vi "Setup DCPower Current for ELOAD.vi"(7 "Channel Groups?":bool, 8 "error in":errorcluster, 9 "Parameters":T1={"Supply"=0.0, "Limit"=0.0, "Aperture Time"=0.0, "Settling Time"=0.0, "Sense"=1008, "Transient Response"=1041} {"Transient Response" items=["Slow"=1041, "Normal"=1038, "Fast"=1039, "Custom"=1042]; "Sense" items=["Local"=1008, "Remote"=1009]}, 10 "Channel List":string, 11 "DCPower Handle In":refnum<k15>) -> (0 "error out":errorcluster, 3 "DCPower Handle Out":refnum<k15>)   [LabVIEW 2021, in "PMIC Common.lvlib"]
uses:
  PMIC Common.lvlib
  DCPower Parameters.ctl
  <instrlib>/niDCPower/nidcpower.llb/niDCPower Output Function.ctl
  <instrlib>/niDCPower/nidcpower.llb/niDCPower Source Mode.ctl
  <instrlib>/niDCPower/nidcpower.llb/niDCPower Wait For Event - Event.ctl
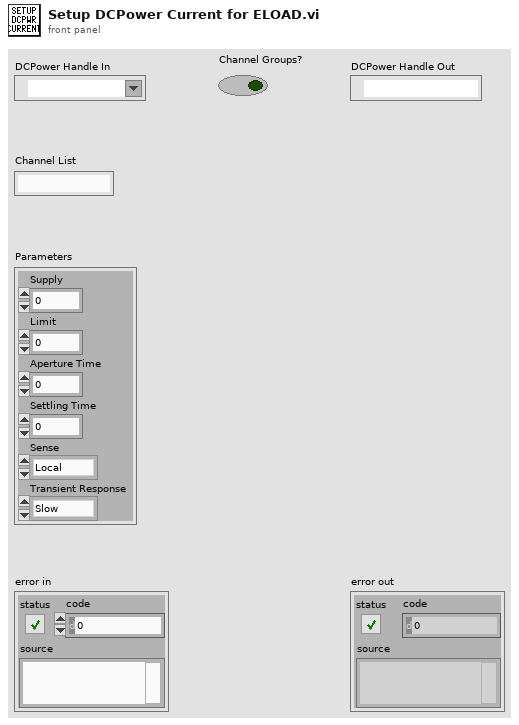
[diagram p1: front panel]
types:
  T1 = typedef "PMIC Common.lvlib/DCPower Parameters.ctl" = cluster{"Supply":dbl, "Limit":dbl, "Aperture Time":dbl, "Settling Time":dbl, "Sense":i32, "Transient Response":i32}
  T2 = typedef "niDCPower Source Mode.ctl" = i32
  T3 = typedef "niDCPower Output Function.ctl" = i32
  T4 = typedef "niDCPower Wait For Event - Event.ctl" = i32
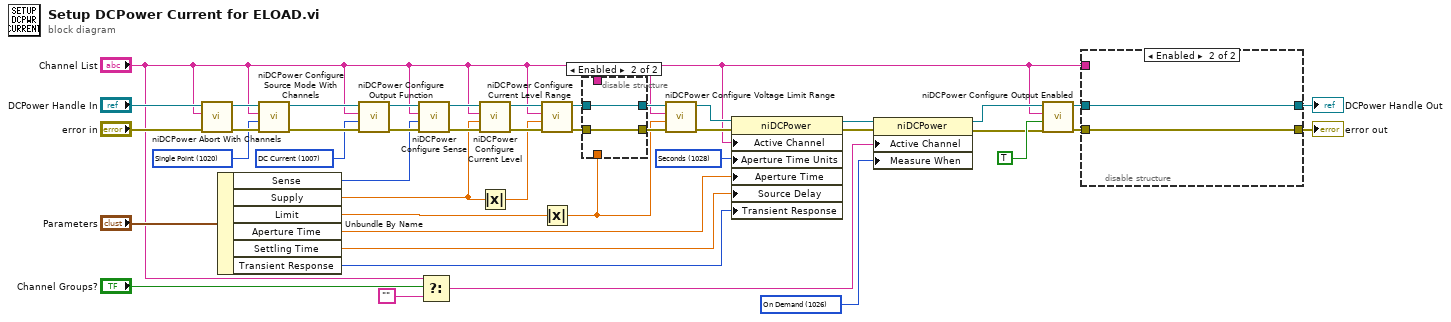
[diagram p0: block diagram]
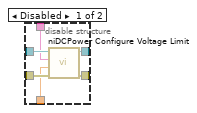
[diagram p2: hidden frame]
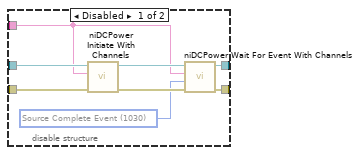
[diagram p3: hidden frame]
diagram:
  w15 = 1026 items=["Automatically after Source Complete"=1025, "On Demand"=1026, "On Measure Trigger"=1027] ("Measurement:Advanced:Measure When")
  w31 = T2 1020 items=["Single Point"=1020, "Sequence"=1021] ("source mode")
  w35 = 1028 items=["Seconds"=1028, "Power Line Cycles"=1029] ("Measurement:Aperture Time Units")
  w1 = T3 1007 items=["DC Voltage"=1006, "DC Current"=1007, "Pulse Voltage"=1049, "Pulse Current"=1050] ("output function")
  n1 = call <instrlib>:"niDCPower Abort With Channels.vi"("error in (no error)"="error in", "channel name"="Channel List", "instrument handle"="DCPower Handle In") -> ("error out"=w33:errorcluster, "instrument handle out"=w44:refnum<k15>)  [unwired: 7 in]
  n2 = Unbundle By Name("Parameters") -> ("Sense"=w8:i32, "Supply"=w7:dbl, "Limit"=w6:dbl, "Aperture Time"=w5:dbl, "Settling Time"=w4:dbl, "Transient Response"=w3:i32)
  n3 = call <instrlib>:"niDCPower Configure Source Mode With Channels.vi"("error in (no error)"=w33, "source mode"=w31, "channel name"="Channel List", "instrument handle"=w44) -> ("error out"=w32:errorcluster, "instrument handle out"=w34:refnum<k15>)  [unwired: 6 in]
  n4 = call <instrlib>:"niDCPower Configure Output Function.vi"("error in (no error)"=w32, "output function"=w1, "channel name"="Channel List", "instrument handle"=w34) -> ("error out"=w26:errorcluster, "instrument handle out"=w25:refnum<k15>)  [unwired: 6 in]
  n5 = call <instrlib>:"niDCPower Configure Sense.vi"("error in (no error)"=w26, "sense"=w8, "channel name"="Channel List", "instrument handle"=w25) -> ("error out"=w23:errorcluster, "instrument handle out"=w24:refnum<k15>)  [unwired: 6 in]
  n6 = Select(t="Channel List", s="Channel Groups?", f="") -> (s? t:f=w16:string)
  n7 = call <instrlib>:"niDCPower Configure Current Level.vi"("error in (no error)"=w23, "current level"=w7, "channel name"="Channel List", "instrument handle"=w24) -> ("error out"=w43:errorcluster, "instrument handle out"=w42:refnum<k15>)  [unwired: 6 in]
  n8 = Absolute Value(x=w7) -> (abs(x)=w22:dbl)
  n9 = call <instrlib>:"niDCPower Configure Current Level Range.vi"("error in (no error)"=w43, "current level range"=w22, "channel name"="Channel List", "instrument handle"=w42) -> ("error out"=w39:errorcluster, "instrument handle out"=w38:refnum<k15>)  [unwired: 6 in]
  n10 = Absolute Value(x=w6) -> (abs(x)=w27:dbl)
  n11 = disable-structure shown="Enabled" {
    disable-tunnel: [w50 w51] -> w41
    disable-tunnel: [w49 w52] -> w40
    disable-tunnel: w39 -> [w48 w51]
    disable-tunnel: w38 -> [w47 w52]
    disable-tunnel: w27 -> [w46 _]
    disable-tunnel: "Channel List" -> [w45 _]
    frame Disabled {
      n12 = call <instrlib>:"niDCPower Configure Voltage Limit.vi"("error in (no error)"=w48, "voltage limit"=w46, "channel name"=w45, "instrument handle"=w47) -> ("error out"=w50:errorcluster, "instrument handle out"=w49:refnum<k15>)  [unwired: 6 in]
    }
    frame Enabled {
    }
  }
  n13 = call <instrlib>:"niDCPower Configure Voltage Limit Range.vi"("error in (no error)"=w41, "voltage limit range"=w27, "channel name"="Channel List", "instrument handle"=w40) -> ("error out"=w36:errorcluster, "instrument handle out"=w37:refnum<k15>)  [unwired: 6 in]
  n14 = property class="niDCPower"(reference=w37, error in=w36, "Active Channel"="Channel List", "Aperture Time Units"=w35, "Aperture Time"=w5, "Source Delay"=w4, "Transient Response"=w3) -> (reference out=w19:refnum<k15>, error out=w21:errorcluster)
  n15 = property class="niDCPower"(reference=w19, error in=w21, "Active Channel"=w16, "Measure When"=w15) -> (reference out=w20:refnum<k15>, error out=w18:errorcluster)
  n16 = call <instrlib>:"niDCPower Configure Output Enabled.vi"("error in (no error)"=w18, "output enabled"=TRUE, "channel name"="Channel List", "instrument handle"=w20) -> ("error out"=w30:errorcluster, "instrument handle out"=w29:refnum<k15>)  [unwired: 6 in]
  n17 = disable-structure shown="Enabled" {
    disable-tunnel: w30 -> [w57 w61]
    disable-tunnel: w29 -> [w56 w62]
    disable-tunnel: [w55 w61] -> w11
    disable-tunnel: [w54 w62] -> w10
    disable-tunnel: "Channel List" -> [w53 _]
    frame Disabled {
      w58 = T4 1030 items=["Source Complete Event"=1030, "Measure Complete Event"=1031, "Sequence Iteration Complete Event"=1032, "Sequence Engine Done Event"=1033, "Pulse Complete Event"=1051, "Ready For Pulse Trigger Event"=1052] ("event")
      n18 = call <instrlib>:"niDCPower Initiate With Channels.vi"("error in (no error)"=w57, "channel name"=w53, "instrument handle"=w56) -> ("error out"=w59:errorcluster, "instrument handle out"=w60:refnum<k15>)  [unwired: 7 in]
      n19 = call <instrlib>:"niDCPower Wait For Event With Channels.vi"("error in (no error)"=w59, "event"=w58, "channel name"=w53, "instrument handle"=w60) -> ("error out"=w55:errorcluster, "instrument handle out"=w54:refnum<k15>)  [unwired: 6 in]
    }
    frame Enabled {
    }
  }
  "error out" <- w11
  "DCPower Handle Out" <- w10
